vi "Feeder_Test.vi"(11 "Joystick Controls":T1) -> ()   [LabVIEW 2020]
uses:
  Utility VIs/Joystick_Controls.ctl
  Systems/Feeder/Feeder_Cluster.ctl
  Systems/Feeder/Feeder_Motor_global.vi
panel:
  in  "funnel_throttle":dbl=1.0
  in  "Magazine_Power":dbl=0.5
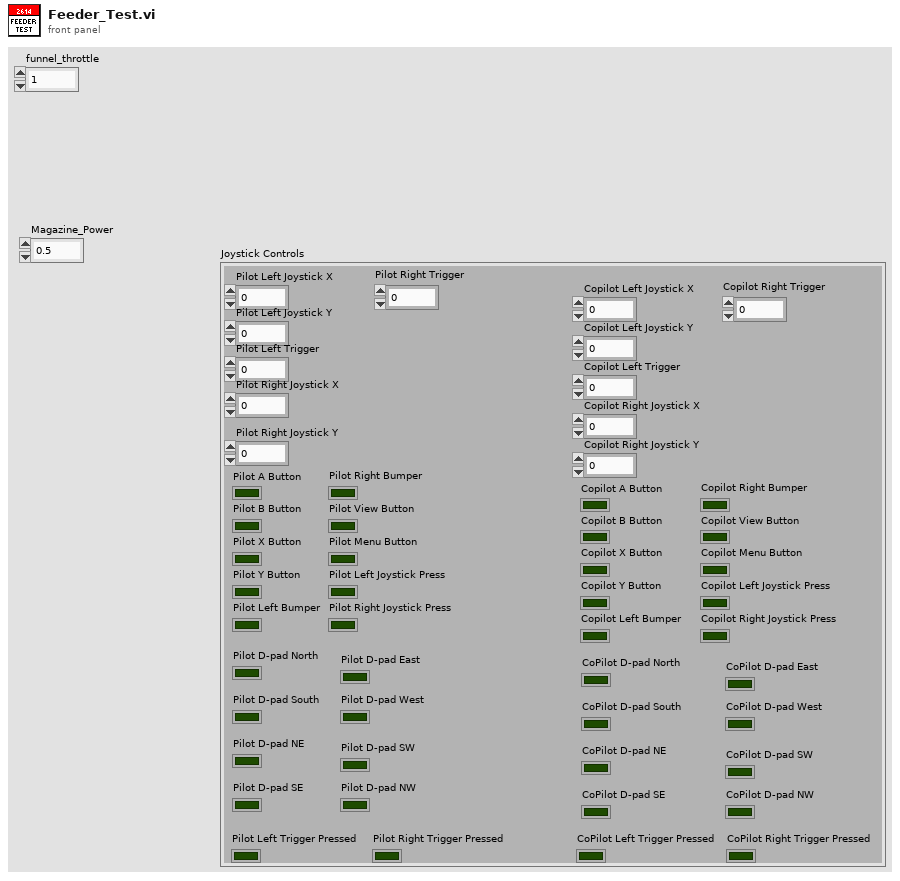
[diagram p1: front panel]
types:
  T1 = typedef "Joystick_Controls.ctl" = cluster{"Pilot Left Joystick X":dbl, "Pilot Left Joystick Y":dbl, "Pilot A Button":bool, "Pilot B Button":bool, "Pilot X Button":bool, "Pilot Y Button":bool, "Pilot Left Bumper":bool, "Pilot Right Bumper":bool, "Pilot View Button":bool, "Pilot Menu Button":bool, "Pilot Left Joystick Press":bool, "Pilot Right Joystick Press":bool, "Pilot Left Trigger":dbl, "Pilot Right Joystick X":dbl, "Pilot Right Joystick Y":dbl, "Pilot Right Trigger":dbl, "Copilot Left Joystick X":dbl, "Copilot Left Joystick Y":dbl, "Copilot A Button":bool, "Copilot B Button":bool, "Copilot X Button":bool, "Copilot Y Button":bool, "Copilot Left Bumper":bool, "Copilot Right Bumper":bool, "Copilot View Button":bool, "Copilot Menu Button":bool, "Copilot Left Joystick Press":bool, "Copilot Right Joystick Press":bool, "Copilot Left Trigger":dbl, "Copilot Right Joystick X":dbl, "Copilot Right Joystick Y":dbl, "Copilot Right Trigger":dbl, "Pilot D-pad North":bool, "Pilot D-pad South":bool, "Pilot D-pad East":bool, "Pilot D-pad West":bool, "Pilot D-pad NE ":bool, "Pilot D-pad SE":bool, "Pilot D-pad SW":bool, "Pilot D-pad NW":bool, "CoPilot D-pad North":bool, "CoPilot D-pad South":bool, "CoPilot D-pad East":bool, "CoPilot D-pad West":bool, "CoPilot D-pad NE":bool, "CoPilot D-pad SE":bool, "CoPilot D-pad SW":bool, "CoPilot D-pad NW":bool, "Pilot Left Trigger Pressed":bool, "Pilot Right Trigger Pressed":bool, "CoPilot Left Trigger Pressed":bool, "CoPilot Right Trigger Pressed":bool}
  T2 = typedef "Feeder_Cluster.ctl" = cluster{"Firing":bool, "Load":bool, "Magazine_%Vbus":dbl, "Funnel_%Vbus":dbl, "Intake_%Vbus":dbl, "Manual_Extend":bool}
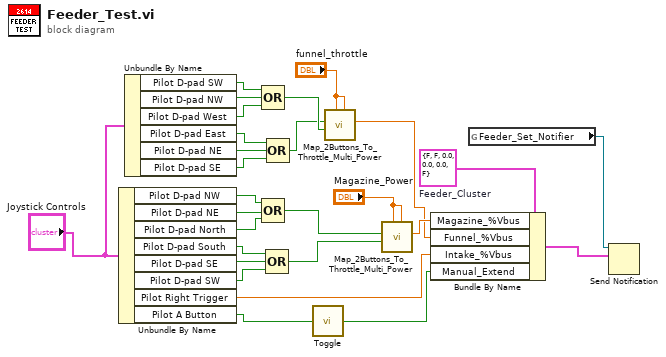
[diagram p0: block diagram]
diagram:
  w27 = T2 {"Firing"=FALSE, "Load"=FALSE, "Magazine_%Vbus"=0.0, "Funnel_%Vbus"=0.0, "Intake_%Vbus"=0.0, "Manual_Extend"=FALSE}  # Feeder_Cluster
  n1 = Unbundle By Name("Joystick Controls") -> ("Pilot D-pad NW"=w24:bool, "Pilot D-pad NE"=w23:bool, "Pilot D-pad North"=w22:bool, "Pilot D-pad South"=w21:bool, "Pilot D-pad SE"=w20:bool, "Pilot D-pad SW"=w19:bool, "Pilot Right Trigger"=w14:dbl, "Pilot A Button"=w2:bool)
  n2 = Unbundle By Name("Joystick Controls") -> ("Pilot D-pad SW"=w13:bool, "Pilot D-pad NW"=w12:bool, "Pilot D-pad West"=w11:bool, "Pilot D-pad East"=w10:bool, "Pilot D-pad NE"=w9:bool, "Pilot D-pad SE"=w8:bool)
  n3 = Compound Arithmetic op=OR(w13, w12, w11) -> (w7:bool)
  n4 = Compound Arithmetic op=OR(w24, w23, w22) -> (w18:bool)
  n5 = Compound Arithmetic op=OR(w21, w20, w19) -> (w17:bool)
  n6 = Compound Arithmetic op=OR(w10, w9, w8) -> (w6:bool)
  n7 = call "Toggle.vi"("Boolean"=w2) -> ("Boolean Out"=w1:bool)
  n8 = call "Map_2Buttons_To_Throttle_Multi_Power.vi"("Power_Down"="funnel_throttle", "Power_Up"="funnel_throttle", "Down"=w7, "Up"=w6) -> ("Throttle"=w3:dbl)  [unwired: 7 in]
  n9 = call "Map_2Buttons_To_Throttle_Multi_Power.vi"("Power_Down"="Magazine_Power", "Power_Up"="Magazine_Power", "Down"=w17, "Up"=w18) -> ("Throttle"=w15:dbl)  [unwired: 7 in]
  n10 = Bundle By Name(cluster=w27, "Magazine_%Vbus"=w15, "Funnel_%Vbus"=w3, "Intake_%Vbus"=w14, "Manual_Extend"=w1) -> (w26:T2)
  n11 = global read "Feeder_Motor_global.vi" "Feeder_Set_Notifier"() -> (w25:refnum<notifier>)
  n12 = Send Notification(notification=w26, notifier=w25) -> ()  [unwired: 1 in, 2 out]
